vi "IMAQ create BG.vi"(11 "Refnum in":T1) -> (3 "Refnum out":T1)   [LabVIEW 2020, in "Point Grey Camera.lvclass"]
uses:
  Point Grey Camera.lvclass
  IMAQ Image.ctl
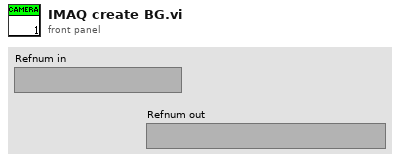
[diagram p1: front panel]
types:
  T1 = typedef "IMAQ Image.ctl" = refnum<image>
  T2 = typedef "Image Type" = u32
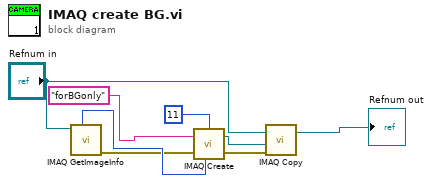
[diagram p0: block diagram]
diagram:
  n1 = call "IMAQ GetImageInfo"("Image"="Refnum in") -> ("error out"=w3:errorcluster, "Image Type"=w7:T2)  [unwired: 3 in, 6 out]
  n2 = call "IMAQ Create"("Border Size"=11, "Image Name"="forBGonly", "Image Type"=w7, "error in (no error)"=w3) -> ("New Image"=w6:T1, "error out"=w4:errorcluster)  [unwired: 1 in]
  n3 = call "IMAQ Copy"("error in (no error)"=w4, "Image Dst"=w6, "Image Src"="Refnum in") -> ("Image Dst Out"=→"Refnum out":T1)  [unwired: 3 in, 1 out]
